vi "Save RSL File.vi"(8 "error in (no error)":errorcluster, 10 "RSL Data":T9={"File Info"={"ID"=1934326086, "Version"=3}, "Parsed Results Data (by VI)"=[], "Parsed Results Data (by Test)"=[], "Raw Results"=[], "Test Config Data"=[], "Numbers"={"Pass"=0, "Fail"=0, "Skipped"=0, "VI not loadable"=0, "Test not loadable"=0, "Test not runnable"=0, "Test error out"=0}, "Tot Time"=0.0, "Timestamp"=0} {"Test Config Data"."Test Ranking" items=["Low", "Normal", "High"]}, 11 "Path":path) -> (0 "error out":errorcluster)   [LabVIEW 2019]
uses:
  <vilib>/addons/analyzer/_vianresshared.llb/VIAnRes Parsed Results Data (by VI).ctl
  <vilib>/addons/analyzer/_vianresshared.llb/VIAnRes Parsed Results Data (by Test).ctl
  <vilib>/addons/analyzer/_analyzerctrls.llb/VIAnCtl Results.ctl
  <vilib>/addons/analyzer/_analyzerctrls.llb/VIAnCtl ResultsData (index).ctl
  <vilib>/addons/analyzer/_analyzerctrls.llb/VIAnCtl ResultStatus.ctl
  <vilib>/addons/analyzer/_analyzerctrls.llb/VIAnCtl Test Config Data.ctl
  <vilib>/addons/analyzer/_analyzerctrls.llb/VIAnCtl TestRanking.ctl
  <vilib>/addons/analyzer/_analyzerctrls.llb/VIAnCtl Config Control Value.ctl
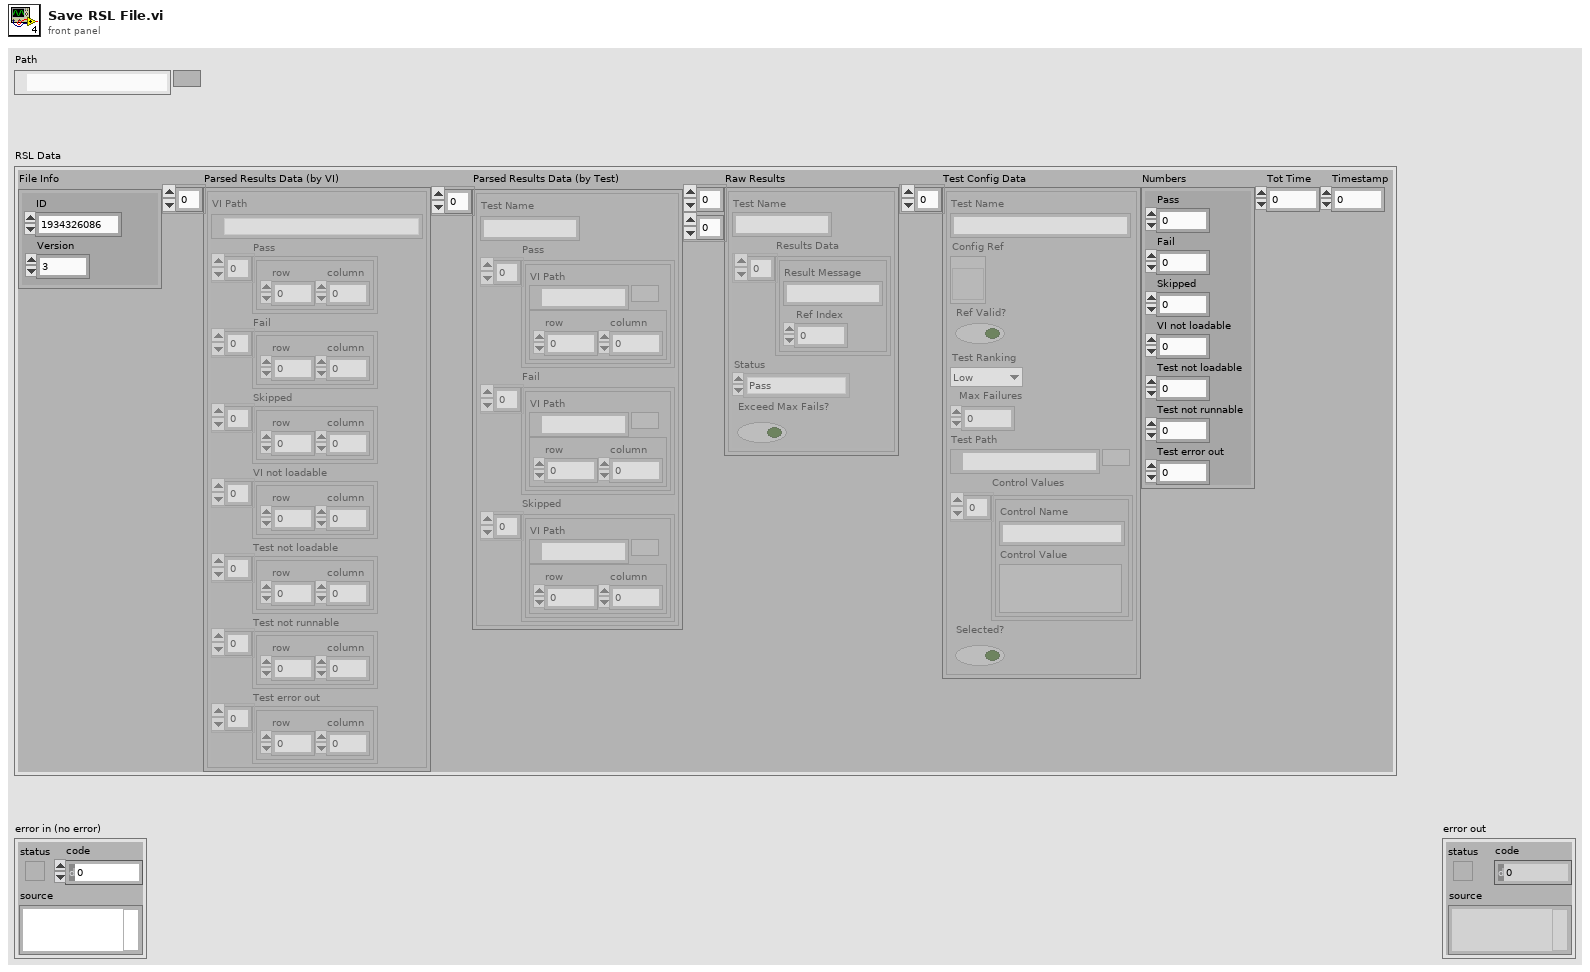
[diagram p1: front panel]
types:
  T1 = typedef "VIAnRes Parsed Results Data (by VI).ctl" = cluster{"VI Path":path, "Pass":cluster{"row":i32, "column":i32}[], "Fail":cluster{"row":i32, "column":i32}[], "Skipped":cluster{"row":i32, "column":i32}[], "VI not loadable":cluster{"row":i32, "column":i32}[], "Test not loadable":cluster{"row":i32, "column":i32}[], "Test not runnable":cluster{"row":i32, "column":i32}[], "Test error out":cluster{"row":i32, "column":i32}[]}
  T2 = typedef "VIAnRes Parsed Results Data (by Test).ctl" = cluster{"Test Name":string, "Pass":cluster{"VI Path":path, "index":cluster{"row":i32, "column":i32}}[], "Fail":cluster{"VI Path":path, "index":cluster{"row":i32, "column":i32}}[], "Skipped":cluster{"VI Path":path, "index":cluster{"row":i32, "column":i32}}[]}
  T3 = typedef "VIAnCtl Results.ctl" = cluster{"Test Name":string, "Results Data":T4[], "Status":T5, "Exceed Max Fails?":bool}
  T4 = typedef "VIAnCtl ResultsData (index).ctl" = cluster{"Result Message":string, "Ref Index":i32}
  T5 = typedef "VIAnCtl ResultStatus.ctl" = enum16{"Pass", "Fail", "Skipped", "VI not loadable", "Test not loadable", "Test not runnable", "Test error out"}
  T6 = typedef "VIAnCtl Test Config Data.ctl" = cluster{"Test Name":string, "Config Ref":refnum<vi>, "Ref Valid?":bool, "Test Ranking":T7, "Max Failures":u32, "Test Path":path, "Control Values":T8[], "Selected?":bool}
  T7 = typedef "VIAnCtl TestRanking.ctl" = u16
  T8 = typedef "VIAnCtl Config Control Value.ctl" = cluster{"Control Name":string, "Control Value":variant}
  T9 = cluster{"File Info":cluster{"ID":i32, "Version":i32}, "Parsed Results Data (by VI)":T1[], "Parsed Results Data (by Test)":T2[], "Raw Results":T3[][], "Test Config Data":T6[], "Numbers":cluster{"Pass":i32, "Fail":i32, "Skipped":i32, "VI not loadable":i32, "Test not loadable":i32, "Test not runnable":i32, "Test error out":i32}, "Tot Time":dbl, "Timestamp":u32}
  T10 = enum16{"open", "replace", "create", "open or create", "replace or create", "replace or create with confirmation"}
  T11 = cluster{"Pass":i32, "Fail":i32, "Skipped":i32, "VI not loadable":i32, "Test not loadable":i32, "Test not runnable":i32, "Test error out":i32}
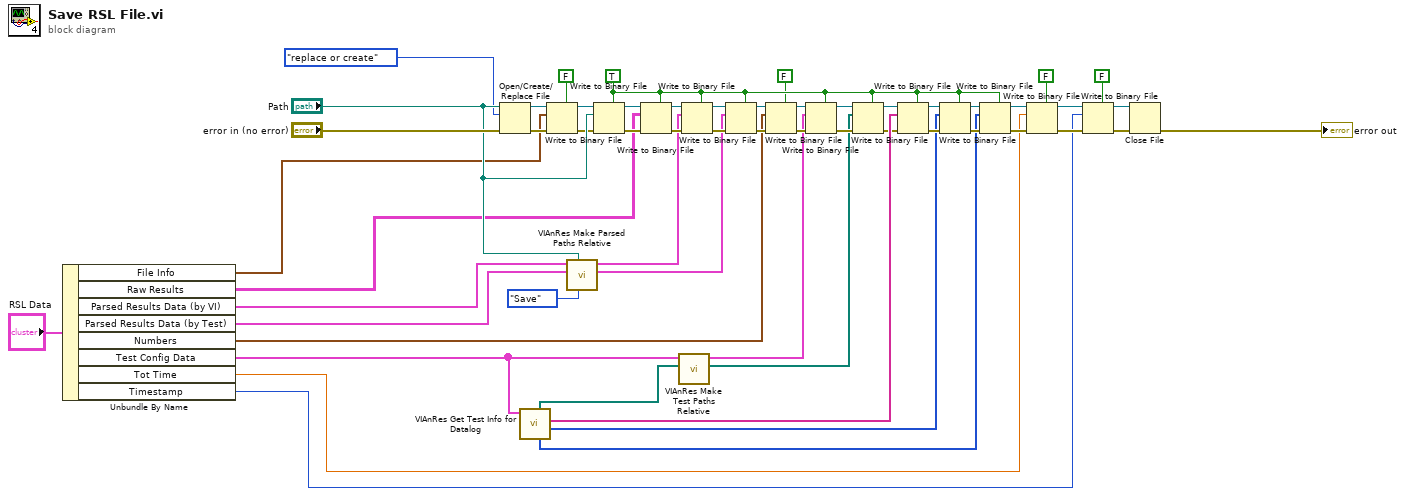
[diagram p0: block diagram]
diagram:
  w21 = TRUE ("header (F)")
  n1 = Unbundle By Name("RSL Data") -> ("File Info"=w3:cluster{"ID":i32, "Version":i32}, "Raw Results"=w2:T3[][], "Parsed Results Data (by VI)"=w4:T1[], "Parsed Results Data (by Test)"=w5:T2[], "Numbers"=w1:T11, "Test Config Data"=w6:T6[], "Tot Time"=w7:dbl, "Timestamp"=w8:u32)
  n2 = Open/Create/Replace File(file path (use dialog)="Path", error in="error in (no error)", operation (0:open)=T10."replace or create") -> (refnum out=w52:refnum<file>, error out=w51:errorcluster)  [unwired: 4 out]
  n3 = call <vilib>:"VIAnRes Get Test Info for Datalog.vi"("Test Config Data"=w6) -> ("Max Failures"=w39:u32[], "Test Tags"=w40:string[], "Test Rankings"=w38:T7[], "Test Paths"=w12:path[])  [unwired: 7 out]
  n4 = Write to Binary File(file (use dialog)=w52, data=w3, error in=w51, 5:FALSE ("prepend array or string size? (T)")) -> (refnum out=w22:refnum<file>, error out=w20:errorcluster)  [unwired: 3 out]
  n5 = call <vilib>:"VIAnRes Make Parsed Paths Relative.vi"("Op"=enum16{"Load", "Save"}."Save", "Current RSL Path"="Path", "Parsed Results Data (by Test) in"=w5, "Parsed Results Data (by VI) in"=w4) -> ("Parsed Results Data (by Test) out"=w23:T2[], "Parsed Results Data (by VI) out"=w24:T1[])  [unwired: 1 in, 5 out]
  n6 = Write to Binary File(file (use dialog)=w22, data="Path", error in=w20, 5:w21) -> (refnum out=w18:refnum<file>, error out=w19:errorcluster)  [unwired: 3 out]
  n7 = Write to Binary File(file (use dialog)=w18, data=w2, error in=w19, 5:w21) -> (refnum out=w30:refnum<file>, error out=w29:errorcluster)  [unwired: 3 out]
  n8 = call <vilib>:"VIAnRes Make Test Paths Relative.vi"("Test Paths in"=w12, "Test Config Data in"=w6) -> ("Test Paths out"=w11:path[], "Test Config Data out"=w31:T6[])  [unwired: 8 in]
  n9 = Write to Binary File(file (use dialog)=w30, data=w24, error in=w29, 5:w21) -> (refnum out=w50:refnum<file>, error out=w49:errorcluster)  [unwired: 3 out]
  n10 = Write to Binary File(file (use dialog)=w50, data=w23, error in=w49, 5:w21) -> (refnum out=w48:refnum<file>, error out=w47:errorcluster)  [unwired: 3 out]
  n11 = Write to Binary File(file (use dialog)=w48, data=w1, error in=w47, 5:FALSE ("prepend array or string size? (T)")) -> (refnum out=w46:refnum<file>, error out=w45:errorcluster)  [unwired: 3 out]
  n12 = Write to Binary File(file (use dialog)=w46, data=w31, error in=w45, 5:w21) -> (refnum out=w28:refnum<file>, error out=w27:errorcluster)  [unwired: 3 out]
  n13 = Write to Binary File(file (use dialog)=w28, data=w11, error in=w27, 5:w21) -> (refnum out=w26:refnum<file>, error out=w25:errorcluster)  [unwired: 3 out]
  n14 = Write to Binary File(file (use dialog)=w26, data=w40, error in=w25, 5:w21) -> (refnum out=w43:refnum<file>, error out=w42:errorcluster)  [unwired: 3 out]
  n15 = Write to Binary File(file (use dialog)=w43, data=w39, error in=w42, 5:w21) -> (refnum out=w44:refnum<file>, error out=w41:errorcluster)  [unwired: 3 out]
  n16 = Write to Binary File(file (use dialog)=w44, data=w38, error in=w41, 5:w21) -> (refnum out=w37:refnum<file>, error out=w36:errorcluster)  [unwired: 3 out]
  n17 = Write to Binary File(file (use dialog)=w37, data=w7, error in=w36, 5:FALSE ("prepend array or string size? (T)")) -> (refnum out=w35:refnum<file>, error out=w34:errorcluster)  [unwired: 3 out]
  n18 = Write to Binary File(file (use dialog)=w35, data=w8, error in=w34, 5:FALSE ("prepend array or string size? (T)")) -> (refnum out=w33:refnum<file>, error out=w32:errorcluster)  [unwired: 3 out]
  n19 = Close File(refnum=w33, error in=w32) -> (error out=→"error out":errorcluster)  [unwired: 1 out]
